vi "USB2XXX_LINEX_ElmosProgramer.vi"() -> ()   [LabVIEW 2010]
panel:
  in  "App File Name":string
  out "Result":bool
  in  "Channel Index":u8(ring) items=["LIN1", "LIN2"]
  in  "Device Index":i32(ring) items=["0", "1", "2", "3", "4", "5"]
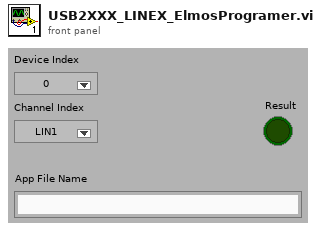
[diagram p1: front panel]
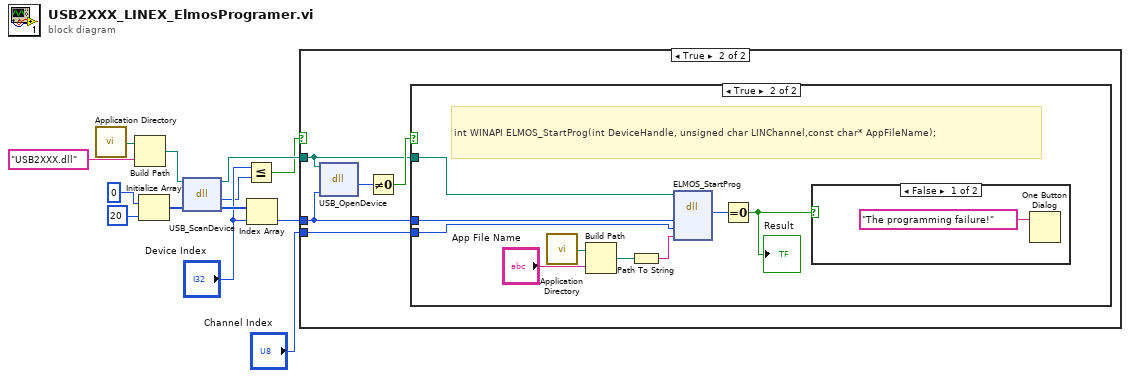
[diagram p0: block diagram]
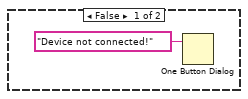
[diagram p2: hidden frame]
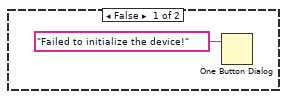
[diagram p3: hidden frame]
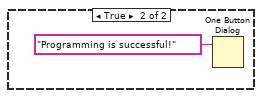
[diagram p4: hidden frame]
diagram:
  n1 = call <vilib>:"Application Directory.vi"() -> ("Application Directory"=w6:path)
  n2 = Build Path(base path=w6, name or relative path="USB2XXX.dll") -> (appended path=w5:path)
  n3 = Initialize Array(0, 20 ("dimension size")) -> (w10:i32[])
  n4 = dll-call lib="E:/OtherWork/STM32/USB2XXX_Example/examples/Labview/PublicFiles/USB2XXX.dll" fn="USB_ScanDevice"(path in=w5, "pDevNum"=w10) -> (path out=w8:path, "return type"=w2:i32, "pDevNum"=w13:i32[])  [unwired: 2 in, 1 out]
  n5 = Less Or Equal?(x="Device Index", y=w2) -> (x <= y?=w4:bool)
  n6 = Index Array(array=w13, index="Device Index") -> (element=w9:i32)
  n7 = case shown="True" w4 {
    tunnel: w9 -> [_ w16]
    tunnel: w8 -> [_ w17]
    tunnel: "Channel Index" -> [_ w15]
    frame False {
      n8 = One Button Dialog(message="Device not connected!") -> ()  [unwired: 1 in, 1 out]
    }
    frame True {
      n9 = dll-call lib="E:/OtherWork/STM32/USB2XXX_Example/examples/Labview/PublicFiles/USB2XXX.dll" fn="USB_OpenDevice"(path in=w17, "DevIndex"=w16) -> ("return type"=w19:u8)  [unwired: 3 in, 2 out]
      n10 = Not Equal To 0?(x=w19) -> (x != 0?=w18:bool)
      n11 = case shown="True" w18 {
        tunnel: w17 -> [_ w24]
        tunnel: w16 -> [_ w23]
        tunnel: w15 -> [_ w22]
        frame False {
          n12 = One Button Dialog(message="Failed to initialize the device!") -> ()  [unwired: 1 in, 1 out]
        }
        frame True {
          # "int WINAPI ELMOS_StartProg(int DeviceHandle, unsigned char LINChannel,const char* AppFileName);"
          n13 = call <vilib>:"Application Directory.vi"() -> ("Application Directory"=w29:path)
          n14 = Build Path(base path=w29, name or relative path="App File Name") -> (appended path=w28:path)
          n15 = Path To String(path=w28) -> (string=w25:string)
          n16 = dll-call lib="E:/Projects/USB2XXX/trunk/USB2XXX/USB2XXX/vs2019/Release/USB2XXX.*" fn="ELMOS_StartProg"(path in=w24, "DeviceHandle"=w23, "LINChannel"=w22, "AppFileName"=w25) -> ("return type"=w21:i32)  [unwired: 5 in, 2 out]
          n17 = Equal To 0?(x=w21) -> (x = 0?=w27:bool)
          "Result" <- w27
          n18 = case shown="False" w27 {
            frame False {
              n19 = One Button Dialog(message="The programming failure!") -> ()  [unwired: 1 in, 1 out]
            }
            frame True {
              n20 = One Button Dialog(message="Programming is successful!") -> ()  [unwired: 1 in, 1 out]
            }
          }
        }
      }
    }
  }
